vi "NF WF1973_74 TRAC Plot.vi"(0 "VISAsession":refnum<visa-resource-name>, 1 "n(12)":i32=12 min=12 max=19 step=1, 2 "Function(Sin)":u16(ring) items=["Sin", "Sin(x)/x", "Clear"], 5 "Memory No.(0)":u16 max=128 step=1, 7 "Name(USER)":string="USER", 9 "Level":i32(knob)=32767 min=-32767 max=32767 step=1 scale=0.0..32767.0, 11 "Error IN":errorcluster, 12 "Read(F)":bool) -> (4 "CopyVISAsession":refnum<visa-resource-name>, 15 "Error OUT":errorcluster)   [LabVIEW 2010]
panel:
  # "n ="
  # "2"
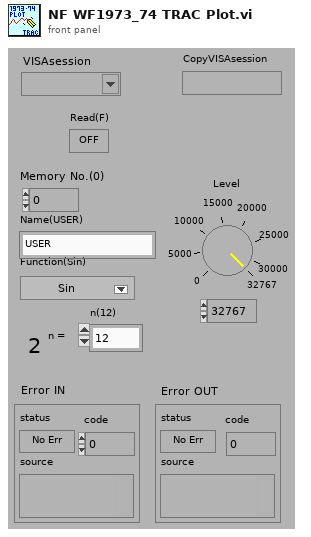
[diagram p1: front panel]
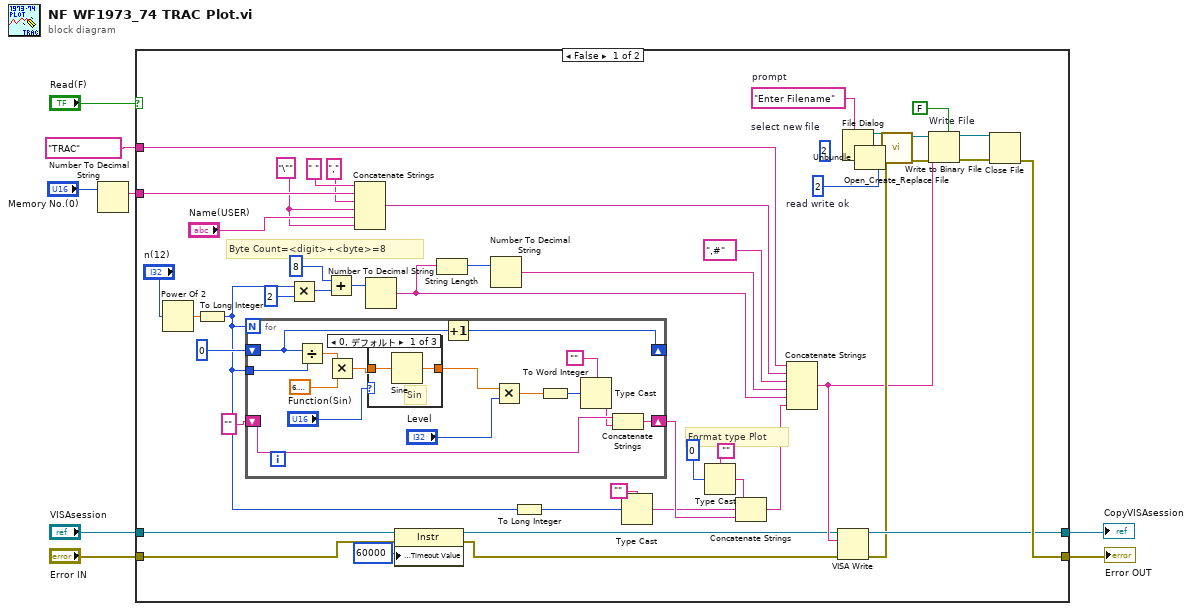
[diagram p0: block diagram]
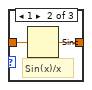
[diagram p2: hidden frame]
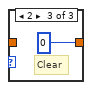
[diagram p3: hidden frame]
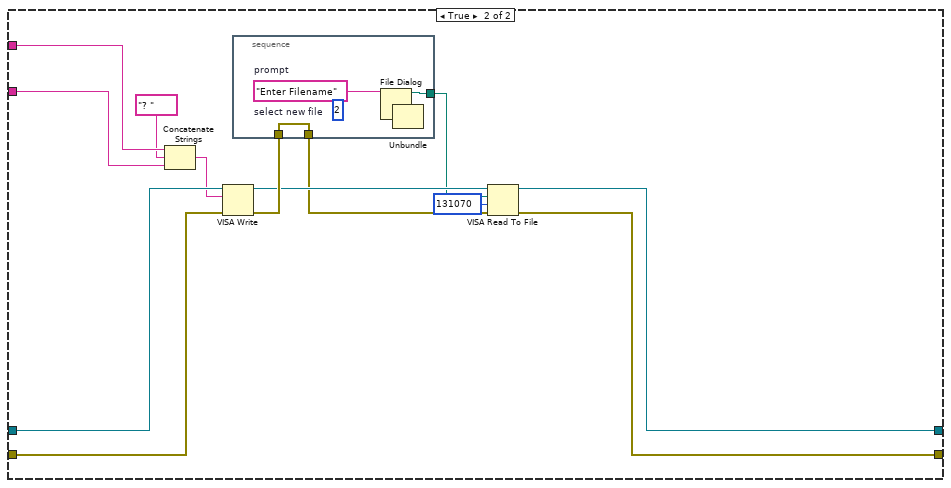
[diagram p4: hidden frame]
diagram:
  n1 = Number To Decimal String(number="Memory No.(0)") -> (decimal integer string=w1:string)  [unwired: 1 in]
  n2 = case shown="FALSE" "Read(F)" {
    tunnel: [w44 w75] -> w8
    tunnel: [w46 w80] -> w7
    tunnel: "VISAsession" -> [w30 w87]
    tunnel: "Error IN" -> [w28 w86]
    tunnel: "TRAC" -> [w14 w84]
    tunnel: w1 -> [w37 w82]
    frame False {
      w12 = "\""
      w53 = "Enter Filename"  # prompt
      w47 = 2  # read write ok
      (unwired) i16 2  # select new file
      # "Format type Plot"
      # "Byte Count=<digit>+<byte>=8"
      n3 = Power Of 2(x="n(12)") -> (2^x=w26:dbl)
      n4 = To Long Integer(number=w26) -> (32bit integer=w11:i32)
      n5 = for {
        N: w11 -> [_]
        shift-right: [w67] -> _
        shift-left: 0 -> [w68]
        tunnel: w11 -> [w60]
        shift-right: [w65] -> w21
        shift-left: "" -> [w64]
        n6 = Divide(x=w68, y=w60) -> (x/y=w58:dbl)
        n7 = Multiply(x=w58, y=6.283185307179586) -> (x*y=w57:dbl)
        n8 = case shown="0, デフォルト" "Function(Sin)" {
          tunnel: w57 -> [w71 w73 _]
          tunnel: [w70 w72 0] -> w56
          frame 0, Default {
            # "Sin"
            n9 = Sine(x=w71) -> (sin(x)=w70:dbl)
          }
          frame 1 {
            # "Sin(x)/x"
            n10 = Sinc(1:w73) -> (0:w72:dbl)
          }
          frame 2 {
            # "Clear"
          }
        }
        n11 = Increment(x=w68) -> (x+1=w67:i32)
        n12 = Multiply(x=w56, y="Level") -> (x*y=w55:dbl)
        n13 = To Word Integer(number=w55) -> (16bit integer=w61:i16)
        n14 = Type Cast(type="", x=w61) -> (*(type *) &x=w62:string)
        n15 = Concatenate Strings(w64, w62) -> (w65:string)
      }
      n16 = Multiply(x=w11, y=2) -> (x*y=w41:i32)
      n17 = Add(x=8, y=w41) -> (x+y=w39:i32)
      n18 = Concatenate Strings(" ", w37, ",", w12, "Name(USER)", w12) -> (w15:string)
      n19 = Number To Decimal String(number=w39) -> (decimal integer string=w18:string)  [unwired: 1 in]
      n20 = property class="Instr"(reference=w30, error in=w28, "General Settings:Timeout Value"=u32 60000) -> (reference out=w31:refnum<visa-resource-name>, error out=w29:errorcluster)
      n21 = String Length(string=w18) -> (length=w38:i32)
      n22 = Number To Decimal String(number=w38) -> (decimal integer string=w19:string)  [unwired: 1 in]
      n23 = To Long Integer(number=w11) -> (32bit integer=w24:i32)
      n24 = Type Cast(type="", x=w24) -> (*(type *) &x=w16:string)
      n25 = Type Cast(type="", x=0) -> (*(type *) &x=w17:string)
      n26 = Concatenate Strings(w17, w16, w21) -> (w22:string)
      n27 = Concatenate Strings(w14, w15, ",#", w19, w18, w22) -> (w34:string)
      n28 = VISA Write(VISA resource name=w31, write buffer=w34, error in (no error)=w29) -> (VISA resource name out=w44:refnum<visa-resource-name>, error out=w43:errorcluster)  [unwired: 1 out]
      n29 = File Dialog(7:w53) -> (0:w10:errorcluster, 3:w50:path)  [unwired: 6 in, 2 out]
      n30 = Unbundle(w10) -> ()  [unwired: 3 out]
      n31 = call <vilib>:"Open_Create_Replace File.vi"("error in (no error)"=w43, "function (open:0)"=w47, "file path"=w50) -> ("error out"=w48:errorcluster, "refnum"=w49:refnum<file>)  [unwired: 5 in, 2 out]
      n32 = Write to Binary File "Write File"(file (use dialog)=w49, data=w34, error in=w48, 5:FALSE ("配列または文字列サイズを先頭に追加?（T）")) -> (refnum out=w52:refnum<file>, error out=w51:errorcluster)  [unwired: 2 in, 1 out]
      n33 = Close File(refnum=w52, error in=w51) -> (error out=w46:errorcluster)  [unwired: 1 out]
    }
    frame True {
      n34 = Concatenate Strings(w84, "? ", w82) -> (w85:string)
      n35 = VISA Write(VISA resource name=w87, write buffer=w85, error in (no error)=w86) -> (VISA resource name out=w79:refnum<visa-resource-name>, error out=w81:errorcluster)  [unwired: 1 out]
      n36 = stacked-sequence {
        tunnel: [w90] -> w76
        tunnel: w81 -> [w89]
        tunnel: [w89] -> w78
        frame #0 {
          w91 = "Enter Filename"  # prompt
          (unwired) i16 2  # select new file
          n37 = File Dialog(7:w91) -> (0:w88:errorcluster, 3:w90:path)  [unwired: 6 in, 2 out]
          n38 = Unbundle(w88) -> ()  [unwired: 3 out]
        }
      }
      n39 = VISA Read To File(8:w78, 9:u32 131070 ("カウント (1024)"), 10:w76, 11:w79) -> (0:w80:errorcluster, 3:w75:refnum<visa-resource-name>)  [unwired: 1 out]
    }
  }
  "CopyVISAsession" <- w8
  "Error OUT" <- w7
